vi "VII Write Bytes.vi"(4 "Len":u16, 5 "pWriteData":string, 6 "SubAddr":i32, 7 "SlaveAddr":u16, 8 "error in (no error)":errorcluster, 9 "I2CIndex":i32, 10 "DevIndex":i32, 11 "DevType":i32) -> (0 "error out":errorcluster, 3 "function return":i32)   [LabVIEW 2012, in "ControlI2C.lvlib"]
doc: "int __stdcall VII_WriteBytes(int DevType,int DevIndex,int I2CIndex,unsigned short SlaveAddr,int SubAddr,unsigned char *pWriteData,unsigned short Len);"
uses:
  ControlI2C.lvlib
  Ginkgo_Driver.dll
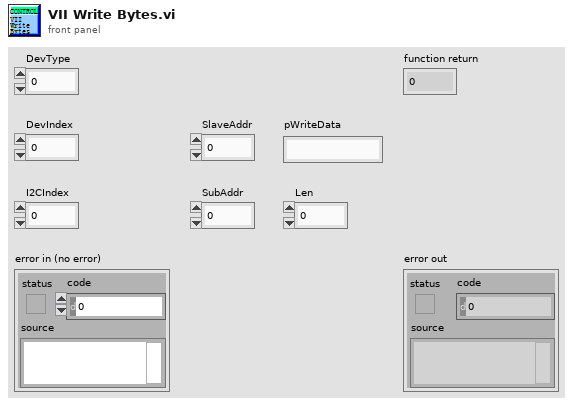
[diagram p1: front panel]
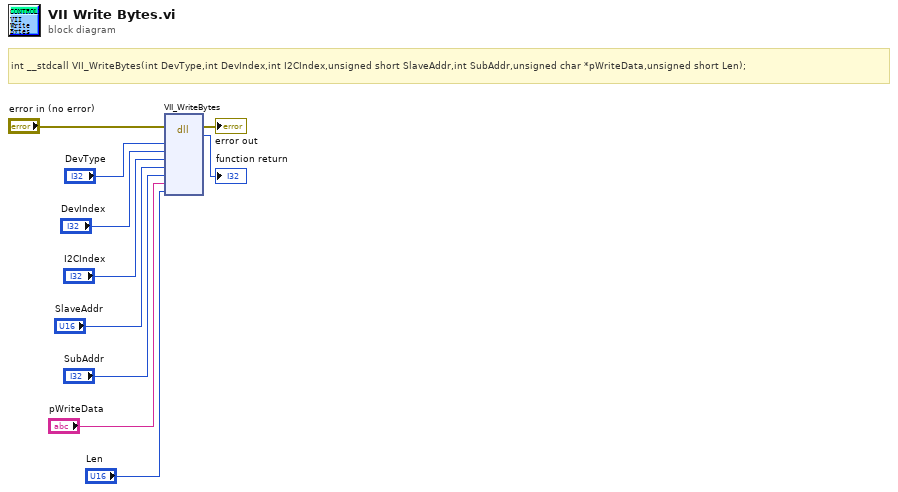
[diagram p0: block diagram]
diagram:
  # "int __stdcall VII_WriteBytes(int DevType,int DevIndex,int I2CIndex,unsigned short SlaveAddr,int SubAddr,unsigned char *pWriteData,unsigned short Len);"
  n1 = dll-call lib="E:/Project/vt_ginkgo/truck/Ginkgo Driver/vs2010/Ginkgo_USB-I2C_API_v2.0.3.0/lib/labview_64bit/ControlI2C/Ginkgo_Driver.*" fn="VII_WriteBytes"(error in="error in (no error)", "DevType"="DevType", "DevIndex"="DevIndex", "I2CIndex"="I2CIndex", "SlaveAddr"="SlaveAddr", "SubAddr"="SubAddr", "pWriteData"="pWriteData", "Len"="Len") -> (error out=→"error out":errorcluster, →"function return":i32)  [unwired: 9 in, 1 out]
